vi "Measurement Logic.vi"() -> ()   [LabVIEW 2021, in "Frequency Response_Audio ADC.lvlib"]
uses:
  Frequency Response_Audio ADC.lvlib
  <vilib>/addons/_NISVFA/_Generation/Signal Generation/SV Discrete Sweep/SV Discrete Sweep.lvclass
  shared/Audio ADC Shared.lvlib
  <vilib>/PDM Acquisition Toolkit/host/Classes/Tasks/PCM Input/PCM Input Task.lvclass
  <vilib>/PDM Acquisition Toolkit/host/Classes/Tasks/PCM Input/Controls/DVR PCM Input Task.ctl
  <vilib>/PDM Acquisition Toolkit/shared/controls/PXI trigger lines.ctl
  <vilib>/PDM Acquisition Toolkit/shared/controls/trigger polarity.ctl
  <vilib>/PDM Acquisition Toolkit/host/API/Controls/PDM Digital Start Trigger Cluster.ctl
  <resource>/objmgr/daqmx.rc
  <vilib>/addons/_NISVFA/_Shared subVIs/Data Objects/Waveforms (DBL)/Waveforms (N Ch).lvclass
  Measurement Results.ctl
  <vilib>/PDM Acquisition Toolkit/host/API/Public/Configure/Triggering/Configure PCM Input Trigger (Digital Edge).vi
  <vilib>/DAQmx/configure/events/hardwareSignals.llb/DAQmx Export Signal (Most Signals).vi
  <vilib>/PDM Acquisition Toolkit/host/API/Public/Start/Start PCM Input Task.vi
  <vilib>/PDM Acquisition Toolkit/host/API/Public/Clear/Clear PCM Input Task.vi
  <vilib>/PDM Acquisition Toolkit/host/API/Public/Read/Read PCM Input Waveform.vi
  <vilib>/DAQmx/write.llb/DAQmx Write (Analog Wfm 1Chan NSamp).vi
  C:/Program Files/National Instruments/LabVIEW 2021/vi.lib/addons/_NISVFA/_Generation/Signal Generation/SV Sinusoid/SV Sinusoid.lvclass
  C:/Program Files/National Instruments/LabVIEW 2021/vi.lib/addons/_NISVFA/_Generation/Signal Generation/SV Function/SV Function.lvclass
  C:/Program Files/National Instruments/LabVIEW 2021/vi.lib/addons/_NISVFA/_Generation/Signal Generation/SV Signal/SV Signal.lvclass
  C:/Program Files/National Instruments/LabVIEW 2021/vi.lib/addons/_NISVFA/_Generation/Signal Generation/SV Discrete Sweep/SV Discrete Sweep.lvclass
  <vilib>/addons/_NISVFA/_Shared subVIs/Data Objects/Waveforms (DBL)/SV Read Next Measurement Data.vi
  Measurement Configuration.ctl
  <vilib>/Plug-In SDKs/Measurements/Measure Call Context/Measure Call Context.lvclass
panel:
  out "measure call context out":refnum<class "Measure Call Context.lvclass">
  in  "measure call context in":refnum<class "Measure Call Context.lvclass">
  out "measurement results":T1
  in  "measurement configuration":T2={"Full scale range"=2.825, "Maximum harmonic"=5, "Analog source resource name"="", "Frequency start"=100.0, "Frequency stop"=20000.0, "Frequency steps"=50, "Frequency spacing"="", "Amplitude"=1.0, "DC Offset"=0.0, "Measurement duration"=0.001, "Measurement cycles"=10, "Settling time"=0.0, "Settling cycles"=0, "Protocol capture resource name"="", "Data line"=0, "Channel"=0, "Sample rate"=12288000.0, "Frame sync edge for channel 0"=1, "Channel count per frame"=2, "Channel length"=32, "Bit depth"=24, "Channel 0 offset"=1, "Endianness"=0, "Data justification"=0, "Frame length"=64, "Frame sync pulse width"=32, "Bit clock edge sync"=1} {"Settling cycles" min=0 max=5 step=1 format="%.3f"}
  out "error out":errorcluster
  in  "error in":errorcluster
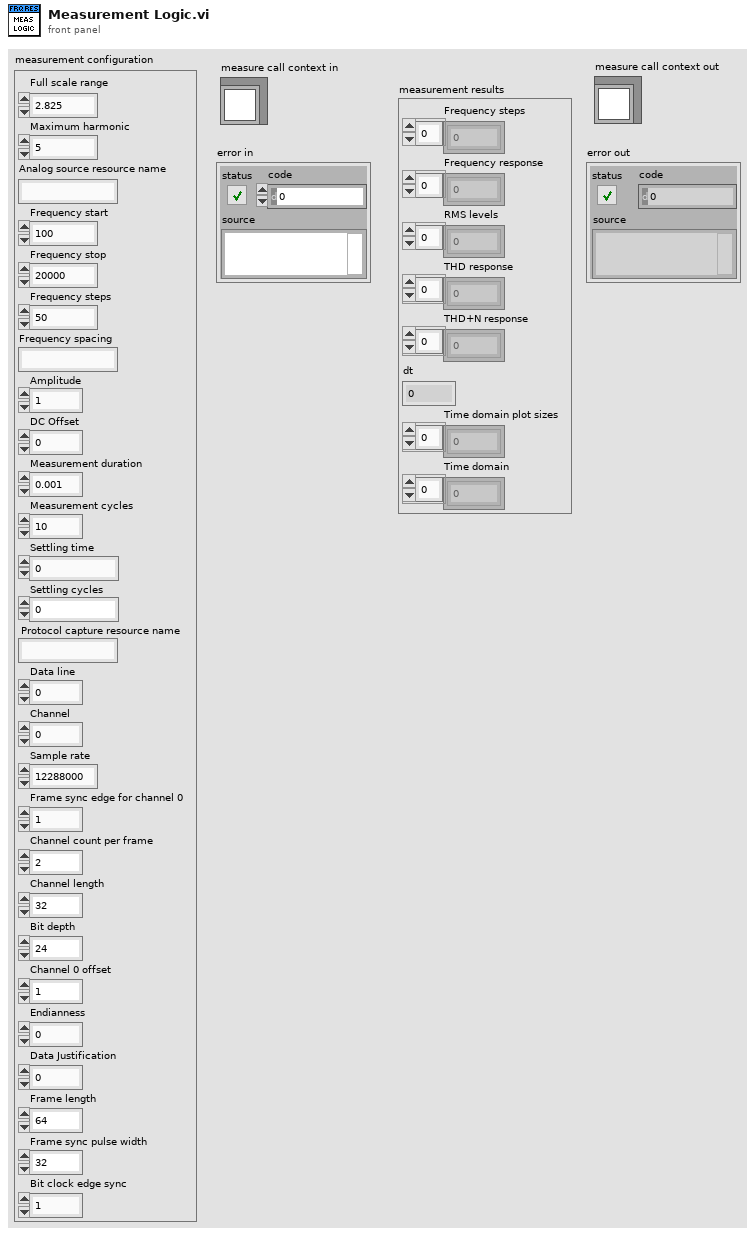
[diagram p1: front panel]
types:
  T1 = typedef "Frequency Response_Audio ADC.lvlib/Measurement Results.ctl" = cluster{"Frequency steps":dbl[], "Frequency response":dbl[], "RMS levels":dbl[], "THD response":dbl[], "THD+N response":dbl[], "dt":dbl, "Time domain plot sizes":i32[], "Time domain":dbl[]}
  T2 = typedef "Frequency Response_Audio ADC.lvlib/Measurement Configuration.ctl" = cluster{"Full scale range":dbl, "Maximum harmonic":i32, "Analog source resource name":string, "Frequency start":dbl, "Frequency stop":dbl, "Frequency steps":i32, "Frequency spacing":string, "Amplitude":dbl, "DC Offset":dbl, "Measurement duration":dbl, "Measurement cycles":i32, "Settling time":dbl, "Settling cycles":i32, "Protocol capture resource name":string, "Data line":u32, "Channel":u32, "Sample rate":dbl, "Frame sync edge for channel 0":u32, "Channel count per frame":u32, "Channel length":u32, "Bit depth":u32, "Channel 0 offset":u32, "Endianness":u32, "Data justification":u32, "Frame length":u32, "Frame sync pulse width":u32, "Bit clock edge sync":u32}
  T3 = typedef "PDM Acquisition Class Library.lvlib/PCM Input Task.lvclass/DVR PCM Input Task.ctl" = refnum<data-value>
  T4 = cluster{"signal configuration":refnum<class "SV Discrete Sweep.lvclass">, "ao task":refnum<k21>, "PDM task":T3, "duration":dbl, "samples":i32, "buffer":refnum<data-value>, "Measurement Results":T1}
  T5 = typedef "PDM Acquisition Toolkit.lvlib/PDM Digital Start Trigger Cluster.ctl" = cluster{"source":T6, "polarity":T7}
  T6 = typedef "PDM Shared.lvlib/PXI trigger lines.ctl" = enum16{"PXI_Trig0", "PXI_Trig1", "PXI_Trig2", "PXI_Trig3", "PXI_Trig4", "PXI_Trig5", "PXI_Trig6", "PXI_Trig7"}
  T7 = typedef "PDM Shared.lvlib/trigger polarity.ctl" = enum16{"Rising Edge", "Falling Edge"}
  T8 = cluster{"measured (s)":dbl[], "maximum (samples)":i32}
  T9 = typedef "audio adc controls.lvlib/Protocol Settings.ctl" = cluster{"Protocol capture resource name":string, "Data line":u16, "Channel":u32, "Clock rate":u32, "Number of words":i32, "Sensitivity":dbl, "Frame sync edge for channel 0":enum32{"Rising", "Falling"}, "Channel count per frame":u8, "Channel length":u16, "Bit depth":u8, "Channel 0 offset":u16, "Endianness":enum32{"MSB First", "LSB First"}, "Data justification":enum32{"Left Justified", "Right Justified"}, "Frame length":u16, "Frame sync pulse width":u16, "Bit clock edge sync":enum32{"Rising", "Falling"}}
  T10 = cluster{"RMS level":dbl, "THD":dbl, "THD+N":dbl, "Frequency":dbl}
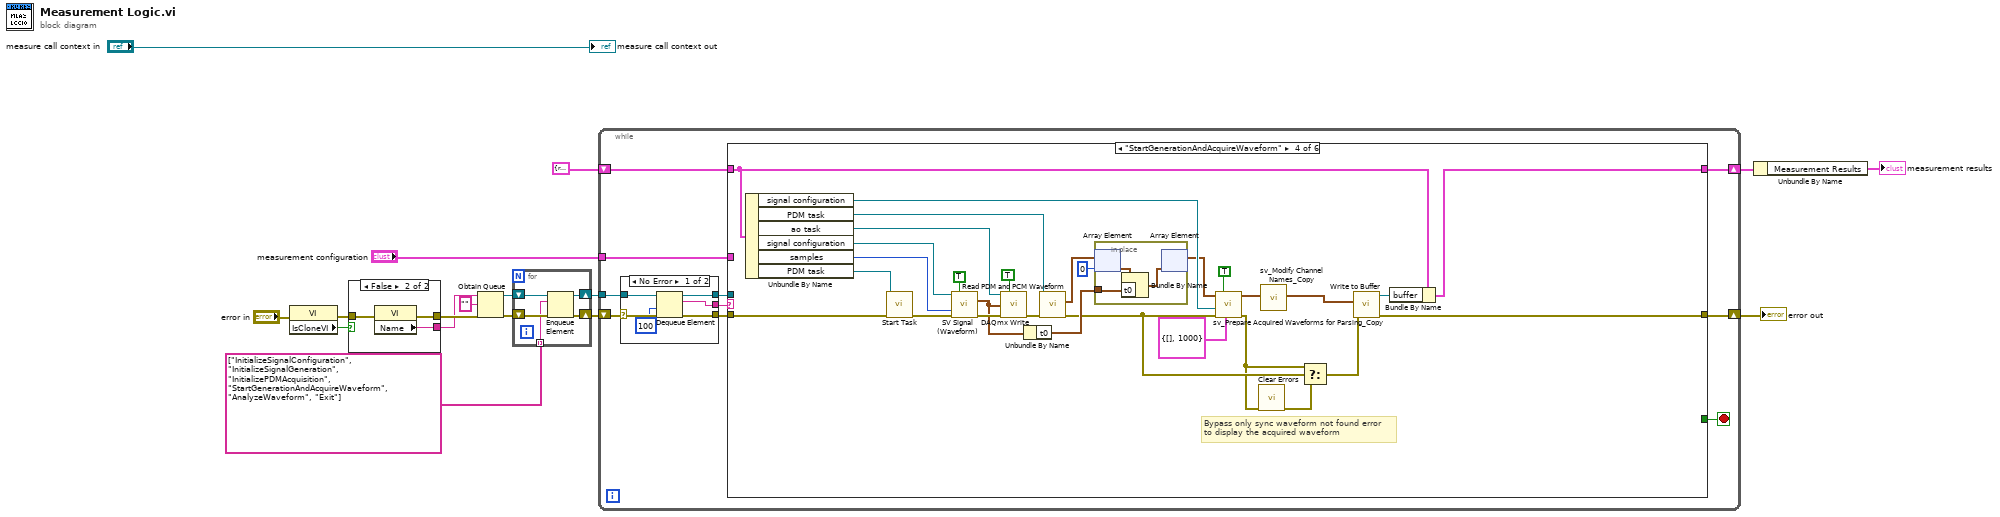
[diagram p0: block diagram]
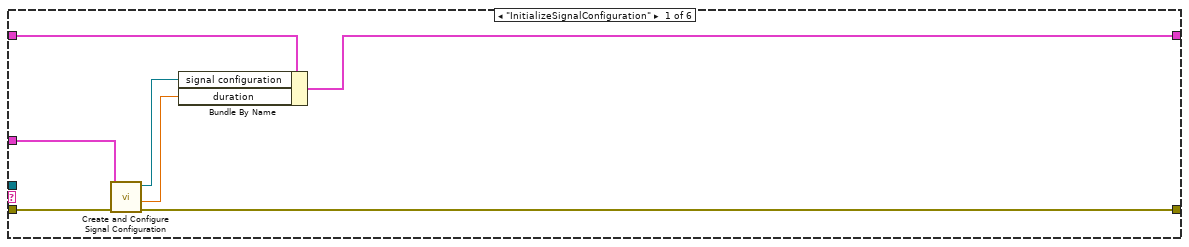
[diagram p2: hidden frame]
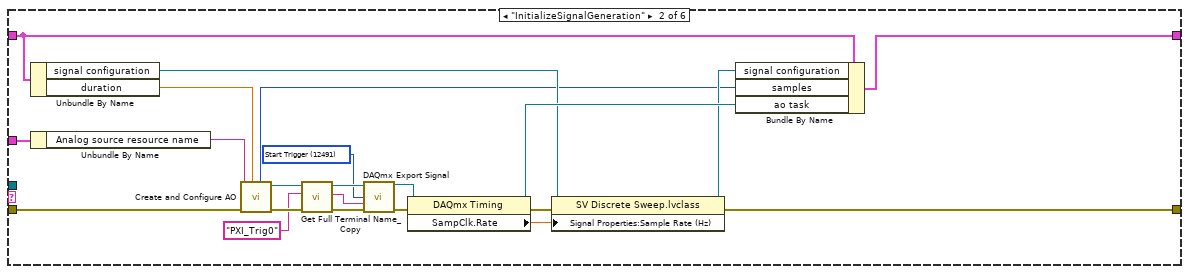
[diagram p3: hidden frame]
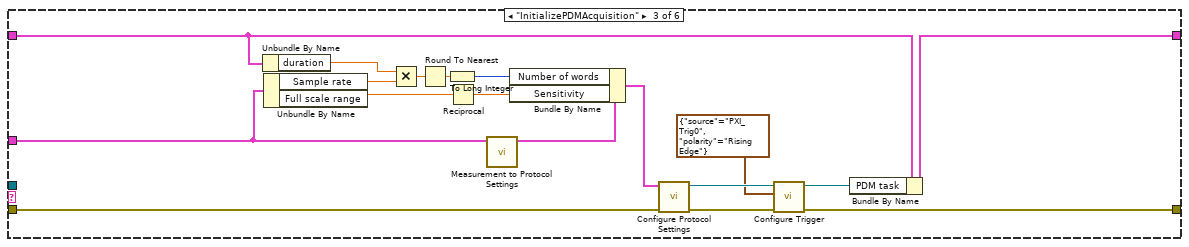
[diagram p4: hidden frame]
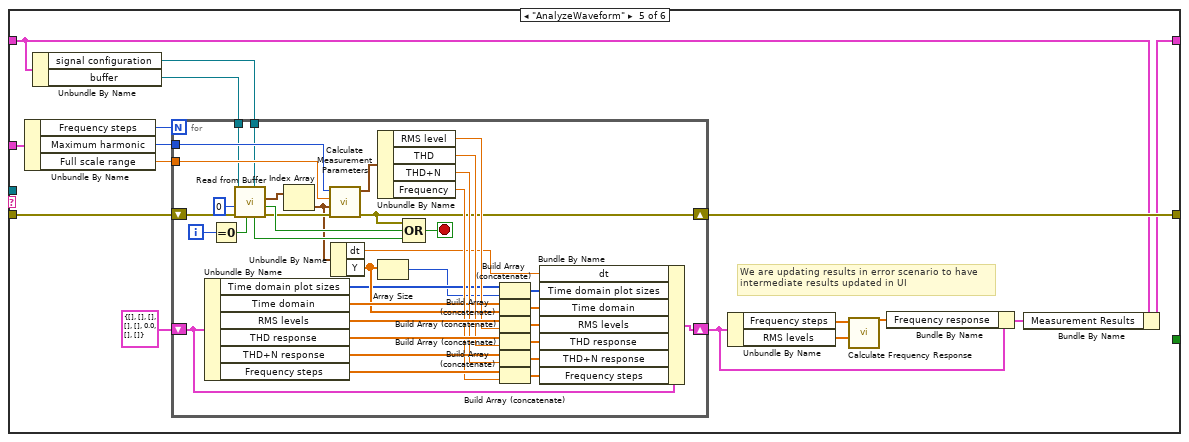
[diagram p5: hidden frame]
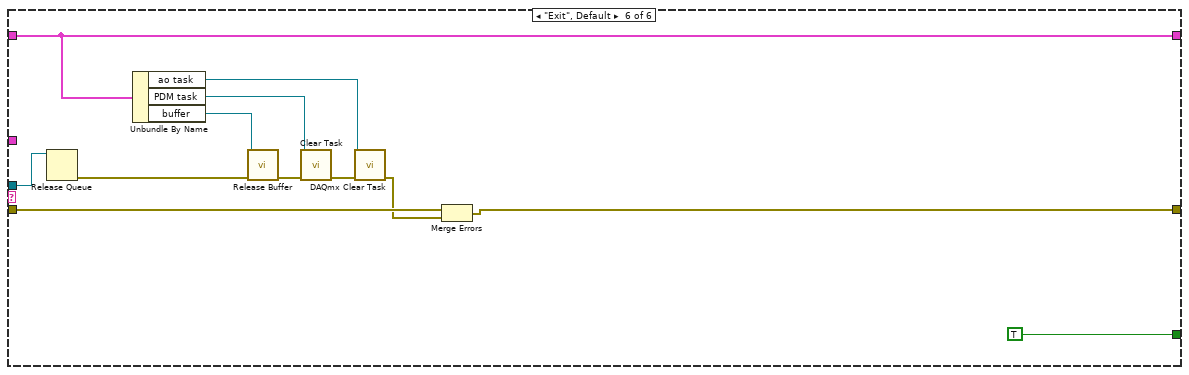
[diagram p6: hidden frame]
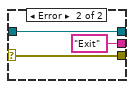
[diagram p7: hidden frame]
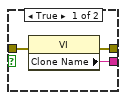
[diagram p8: hidden frame]
diagram:
  n1 = property class="VI"(error in="error in") -> (error out=w13:errorcluster, "IsCloneVI"=w14:bool)  [unwired: 1 in, 1 out]
  n2 = case shown="False" w14 {
    tunnel: [w20 w23] -> w12
    tunnel: [w19 w22] -> w11
    tunnel: w13 -> [w18 w21]
    frame True {
      n3 = property class="VI"(error in=w18) -> (error out=w20:errorcluster, "Clone Name"=w19:string)  [unwired: 1 in, 1 out]
    }
    frame False {
      n4 = property class="VI"(error in=w21) -> (error out=w23:errorcluster, "Name"=w22:string)  [unwired: 1 in, 1 out]
    }
  }
  n5 = Obtain Queue(name (unnamed)=w11, element data type="", error in (no error)=w12) -> (queue out=w15:refnum<queue>, error out=w10:errorcluster)  [unwired: 2 in, 1 out]
  n6 = for {
    shift-right: [w26] -> w7
    shift-left: w15 -> [w28]
    shift-right: [w25] -> w6
    shift-left: w10 -> [w27]
    tunnel: string[] ["InitializeSignalConfiguration", "InitializeSignalGeneration", "InitializePDMAcquisition", "StartGenerationAndAcquireWaveform", "AnalyzeWaveform", "Exit"] ("Step sequence") -> [w24] mode=indexing
    n7 = Enqueue Element(queue=w28, element=w24, error in (no error)=w27) -> (queue out=w26:refnum<queue>, error out=w25:errorcluster)  [unwired: 1 in, 1 out]
  }
  n8 = while {
    tunnel: w7 -> [w38]
    tunnel: "measurement configuration" -> [w33]
    shift-right: [w30] -> w2
    shift-left: T4 {"signal configuration"=refnum, "ao task"="", "PDM task"=refnum, "duration"=0.0, "samples"=0, "buffer"=refnum, "Measurement Results"={"Frequency steps"=[], "Frequency response"=[], "RMS levels"=[], "THD response"=[], "THD+N response"=[], "dt"=0.0, "Time domain plot sizes"=[], "Time domain"=[]}} ("output cluster") -> [w31]
    shift-right: [w29] -> w3
    shift-left: w6 -> [w37]
    stop <- w34 stop-if-true
    n9 = case shown="No Error" w37 {
      selector: w37 -> [w186 w190]
      tunnel: w38 -> [w188 w189]
      tunnel: [w187 "Exit" ("t")] -> w36
      tunnel: [w185 w190] -> w32
      tunnel: [w183 w189] -> w35
      frame No Error {
        n10 = Dequeue Element(queue=w188, timeout in ms (-1)=100, error in (no error)=w186) -> (queue out=w183:refnum<queue>, element=w187:string, error out=w185:errorcluster)  [unwired: 1 out]
      }
      frame Error {
      }
    }
    n11 = case shown="\"StartGenerationAndAcquireWaveform\"" w36 {
      tunnel: w35 -> [_ _ _ _ _ w182]
      tunnel: [_ _ _ _ _ TRUE] -> w34
      tunnel: w33 -> [w44 w67 w68 _ w132 _]
      tunnel: w32 -> [w45 w65 w85 w97 w133 w172]
      tunnel: w31 -> [w43 w64 w81 w99 w127 w180]
      tunnel: [w40 w63 w84 w100 w122 w180] -> w30
      tunnel: [w39 w53 w75 w102 w129 w173] -> w29
      frame "InitializeSignalConfiguration" {
        n12 = call "Create and Configure Signal Configuration.vi"("error in"=w45, "Measurement configuration"=w44) -> ("error out"=w39:errorcluster, "duration"=w41:dbl, "signal configuration"=w42:refnum<class "SV Discrete Sweep.lvclass">)  [unwired: 7 in]
        n13 = Bundle By Name(cluster=w43, "signal configuration"=w42, "duration"=w41) -> (w40:T4)
      }
      frame "InitializeSignalGeneration" {
        w57 = 12491 items=["AI Convert Clock"=12484, "10MHz Reference Clock"=12536, "20MHz Timebase Clock"=12486, "Sample Clock"=12487, "Advance Trigger"=12488, "Reference Trigger"=12490, "Start Trigger"=12491, "Advance Complete Event"=12492, "AI Hold Complete Event"=12493, "Counter Output Event"=12494, "Change Detection Event"=12511, "Watchdog Timer Expired Event"=12512] ("signal")
        n14 = Unbundle By Name(w64) -> ("signal configuration"=w49:refnum<class "SV Discrete Sweep.lvclass">, "duration"=w47:dbl)
        n15 = Unbundle By Name(w67) -> ("Analog source resource name"=w66:string)
        n16 = call "Create and Configure AO.vi"("duration"=w47, "error in"=w65, "AO channel"=w66) -> ("error out"=w62:errorcluster, "AO task"=w51:refnum<k21>, "samples"=w46:i32)  [unwired: 6 in]
        n17 = call "Get Full Terminal Name_Copy.vi"("error in"=w62, "Local Terminal Name"="PXI_Trig0" ("Trigger line"), "task/channels in"=w51) -> ("error out"=w59:errorcluster, "Terminal Name with Device Prefix"=w58:tag, "task out"=w60:refnum<k21>)  [unwired: 6 in]
        n18 = call-poly <vilib>:"DAQmx Export Signal.vi"("task/channels in"=w60, "signal"=w57, "output terminal"=w58, "error in"=w59) -> ("task out"=w52:refnum<k21>, "error out"=w54:errorcluster)  [unwired: 10 in]
        n19 = property class="DAQmx Timing"(reference=w52, error in=w54) -> (reference out=w50:refnum<k21>, error out=w56:errorcluster, "SampClk.Rate"=w55:dbl)
        n20 = property class="SV Discrete Sweep.lvclass"(reference=w49, error in=w56, "Signal Properties:Sample Rate (Hz)"=w55) -> (reference out=w48:refnum<class "SV Discrete Sweep.lvclass">, error out=w53:errorcluster)
        n21 = Bundle By Name(cluster=w64, "signal configuration"=w48, "samples"=w46, "ao task"=w50) -> (w63:T4)
      }
      frame "InitializePDMAcquisition" {
        n22 = Unbundle By Name(w81) -> ("duration"=w80:dbl)
        n23 = Unbundle By Name(w68) -> ("Sample rate"=w71:dbl, "Full scale range"=w70:dbl)
        n24 = Multiply(x=w80, y=w71) -> (x*y=w82:dbl)
        n25 = Round To Nearest(number=w82) -> (nearest integer value=w83:dbl)
        n26 = To Long Integer(number=w83) -> (32bit integer=w74:i32)
        n27 = Reciprocal(x=w70) -> (1/x=w69:dbl)
        n28 = call "Measurement to Protocol Settings.vi"("Measurement Configuration"=w68) -> ("Protocol settings"=w73:T9)  [unwired: 10 in]
        n29 = Bundle By Name(cluster=w73, "Number of words"=w74, "Sensitivity"=w69) -> (w72:T9)
        n30 = call "Configure Protocol Settings.vi"("error in"=w85, "Protocol settings"=w72) -> ("error out"=w78:errorcluster, "PDM task"=w79:T3)  [unwired: 8 in]
        n31 = call-poly <vilib>:"Configure Trigger.vi"("error in"=w78, "trigger configuration"=T5 {"source"=enum."PXI_Trig0", "polarity"=enum."Rising Edge"}, "PCM input task in"=w79) -> ("error out"=w75:errorcluster, "PCM input task out"=w76:T3)  [unwired: 7 in]
        n32 = Bundle By Name(cluster=w81, "PDM task"=w76) -> (w84:T4)
      }
      frame "StartGenerationAndAcquireWaveform" {
        # "Bypass only sync waveform not found error\nto display the acquired waveform"
        n33 = Unbundle By Name(w99) -> ("signal configuration"=w93:refnum<class "SV Discrete Sweep.lvclass">, "PDM task"=w103:T3, "ao task"=w109:refnum<k21>, "signal configuration"=w104:refnum<class "SV Discrete Sweep.lvclass">, "samples"=w105:i32, "PDM task"=w96:T3)
        n34 = call-poly <vilib>:"Start Task.vi"("error in"=w97, "PCM input task in"=w96) -> ("error out"=w98:errorcluster)  [unwired: 8 in, 1 out]
        n35 = call-dynamic "SV Signal (Waveform).vi"("signal configuration"=w104, "reset"=TRUE, "samples"=w105, "error in (no error)"=w98) -> ("output waveform"=w110:waveform(dbl), "error out"=w113:errorcluster)  [unwired: 6 in, 4 out]
        n36 = call-poly <vilib>:"DAQmx Write.vi"("task/channels in"=w109, "auto start"=TRUE, "data"=w110, "error in"=w113) -> ("error out"=w111:errorcluster)  [unwired: 9 in, 2 out]
        n37 = Unbundle By Name(w110) -> ("t0"=w106:timestamp)
        n38 = call-poly <vilib>:"Read PDM and PCM Waveform.vi"("error in"=w111, "PCM input task In"=w103) -> ("error out"=w89:errorcluster, "PCM waveforms"=w108:waveform(dbl)[])  [unwired: 4 in, 4 out]
        n39 = in-place {
          in-place-border: w106 -> [w116]
          n40 = in-place-array #1(w108, 0) -> (w117:waveform(dbl))
          n41 = Bundle By Name(cluster=w117, "t0"=w116) -> (w115:waveform(dbl))
          n42 = in-place-array #1(w115) -> (w92:waveform(dbl)[])  [unwired: 1 out]
        }
        n43 = call "sv_Prepare Acquired Waveforms for Parsing_Copy.vi"("propagation delay"=T8 {"measured (s)"=[], "maximum (samples)"=1000}, "restart (F)"=TRUE, "error in"=w89, "SV Signal"=w93, "acquired channel waveforms"=w92) -> ("error out"=w88:errorcluster, "aligned channel waveforms"=w94:waveform(dbl)[])  [unwired: 4 in, 1 out]
        n44 = call <vilib>:"Clear Errors.vi"("error in (no error)"=w88) -> ("error out"=w87:errorcluster)  [unwired: 5 in, 1 out]
        n45 = call "sv_Modify Channel Names_Copy.vi"("waveforms"=w94) -> ("renamed waveforms"=w95:waveform(dbl)[])  [unwired: 8 in]
        n46 = Select(t=w88, s=w89, f=w87) -> (s? t:f=w86:errorcluster)
        n47 = call <vilib>:"Write to Buffer.vi"("error in (no error)"=w86, "waveforms"=w95) -> ("error out"=w102:errorcluster, "buffer out"=w101:refnum<data-value>)  [unwired: 7 in, 1 out]
        n48 = Bundle By Name(cluster=w99, "buffer"=w101) -> (w100:T4)
      }
      frame "AnalyzeWaveform" {
        # "We are updating results in error scenario to have\nintermediate results updated in UI"
        n49 = Unbundle By Name(w132) -> ("Frequency steps"=w128:i32, "Maximum harmonic"=w130:i32, "Full scale range"=w131:dbl)
        n50 = Unbundle By Name(w127) -> ("signal configuration"=w125:refnum<class "SV Discrete Sweep.lvclass">, "buffer"=w126:refnum<data-value>)
        n51 = for {
          N: w128 -> [_]
          tunnel: w131 -> [w170]
          tunnel: w130 -> [w169]
          shift-right: [w143] -> w129
          shift-left: w133 -> [w168]
          tunnel: w126 -> [w165]
          tunnel: w125 -> [w163]
          shift-right: [w147] -> w123
          shift-left: T1 {"Frequency steps"=[], "Frequency response"=[], "RMS levels"=[], "THD response"=[], "THD+N response"=[], "dt"=0.0, "Time domain plot sizes"=[], "Time domain"=[]} ("Measurement Results") -> [w152]
          i -> [w167]
          stop <- w142 stop-if-true
          n52 = Unbundle By Name(w152) -> ("Time domain plot sizes"=w137:i32[], "Time domain"=w140:dbl[], "RMS levels"=w160:dbl[], "THD response"=w158:dbl[], "THD+N response"=w156:dbl[], "Frequency steps"=w154:dbl[])
          n53 = Equal To 0?(x=w167) -> (x = 0?=w166:bool)
          n54 = call-poly <vilib>:"Read from Buffer.vi"("test signal configuration"=w163, "reset start (F)"=w166, "error in (no error)"=w168, "timeout (1000 ms)"=0, "buffer"=w165) -> ("error out"=w144:errorcluster, "end of buffer"=w146:bool, "waveforms subset"=w162:waveform(dbl)[], "done"=w145:bool)  [unwired: 2 in, 1 out]
          n55 = Index Array(array=w162) -> (element=w141:waveform(dbl))  [unwired: 1 in]
          n56 = call "Calculate Measurement Parameters.vi"("error in"=w144, "scaled signal in [EU]"=w141, "Full scale range"=w170, "Maximum harmonic"=w169) -> ("error out"=w143:errorcluster, "Meas results"=w161:T10)  [unwired: 6 in]
          n57 = Unbundle By Name(w141) -> ("dt"=w134:dbl, "Y"=w138:dbl[])
          n58 = Unbundle By Name(w161) -> ("RMS level"=w159:dbl, "THD"=w157:dbl, "THD+N"=w155:dbl, "Frequency"=w153:dbl)
          n59 = Array Size(array=w138) -> (size(s)=w136:i32)
          n60 = Compound Arithmetic op=OR(w143, w146, w145) -> (w142:bool)
          n61 = Build Array (concatenate)(w137, w136) -> (w135:i32[])
          n62 = Build Array (concatenate)(w140, w138) -> (w139:dbl[])
          n63 = Build Array (concatenate)(w160, w159) -> (w151:dbl[])
          n64 = Build Array (concatenate)(w158, w157) -> (w150:dbl[])
          n65 = Build Array (concatenate)(w156, w155) -> (w149:dbl[])
          n66 = Build Array (concatenate)(w154, w153) -> (w148:dbl[])
          n67 = Bundle By Name(cluster=w152, "dt"=w134, "Time domain plot sizes"=w135, "Time domain"=w139, "RMS levels"=w151, "THD response"=w150, "THD+N response"=w149, "Frequency steps"=w148) -> (w147:T1)
        }
        n68 = Unbundle By Name(w123) -> ("Frequency steps"=w124:dbl[], "RMS levels"=w119:dbl[])
        n69 = call "Calculate Frequency Response.vi"("Amplitudes"=w119, "Frequencies"=w124) -> ("Frequency response @ 1KHz"=w118:dbl[])  [unwired: 9 in]
        n70 = Bundle By Name(cluster=w123, "Frequency response"=w118) -> (w121:T1)
        n71 = Bundle By Name(cluster=w127, "Measurement Results"=w121) -> (w122:T4)
      }
      frame "Exit", Default {
        n72 = Release Queue(queue=w182) -> (error out=w178:errorcluster)  [unwired: 2 in, 2 out]
        n73 = Unbundle By Name(w180) -> ("ao task"=w174:refnum<k21>, "PDM task"=w176:T3, "buffer"=w179:refnum<data-value>)
        n74 = call <vilib>:"Release Buffer.vi"("error in (no error)"=w178, "buffer"=w179) -> ("error out"=w177:errorcluster)  [unwired: 9 in]
        n75 = call-poly <vilib>:"Clear Task.vi"("error in"=w177, "PCM input task in"=w176) -> ("error out"=w175:errorcluster)  [unwired: 9 in]
        n76 = call <vilib>:"DAQmx Clear Task.vi"("task in"=w174, "error in"=w175) -> ("error out"=w171:errorcluster)  [unwired: 13 in]
        n77 = Merge Errors(w172, w171) -> (w173:errorcluster)
      }
    }
  }
  "error out" <- w3
  n78 = Unbundle By Name(w2) -> ("Measurement Results"=→"measurement results":T1)
  "measure call context out" <- "measure call context in"
